vi "Set Topic Value.vi"(8 "error in (no error)":errorcluster, 9 "Value":variant, 10 "Topic":string, 11 "Communications in":refnum<class "Communications.lvclass">) -> (0 "error out":errorcluster, 2 "replaced":bool, 3 "Communications out":refnum<class "Communications.lvclass">)   [LabVIEW 2019, in "Communications.lvclass"]
uses:
  Communications.lvclass
  Communications.lvclass/Communications.ctl
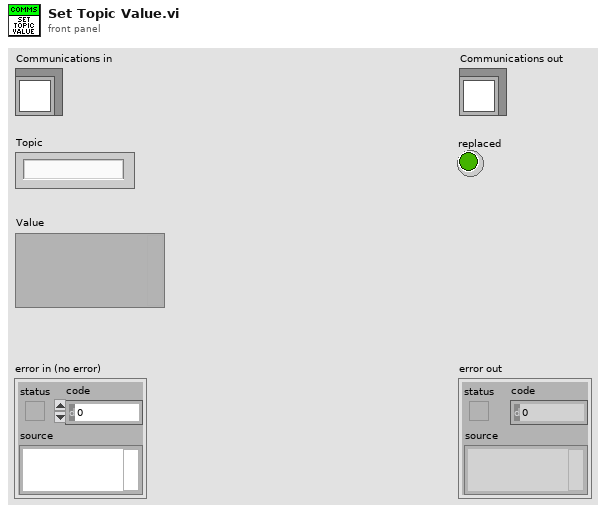
[diagram p1: front panel]
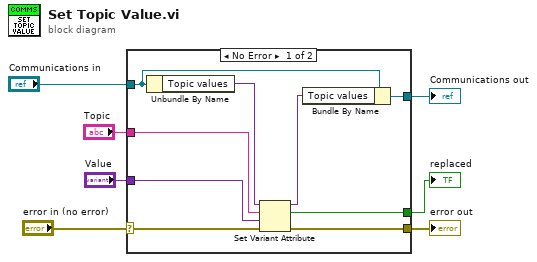
[diagram p0: block diagram]
diagram:
  n1 = case shown="No Error" "error in (no error)" {
    selector: "error in (no error)" -> [w14 w18]
    tunnel: [w11 w18] -> w6
    tunnel: [w10 w17] -> w4
    tunnel: "Communications in" -> [w16 w17]
    tunnel: "Value" -> [w13 _]
    tunnel: "Topic" -> [w12 _]
    tunnel: [w8 _] -> w1
    frame No Error {
      n2 = Unbundle By Name(w16) -> ("Topic values"=w15:variant)
      n3 = Set Variant Attribute(Variant=w15, name=w12, value=w13, error in=w14) -> (Variant out=w9:variant, replaced=w8:bool, error out=w11:errorcluster)
      n4 = Bundle By Name(cluster=w16, "Topic values"=w9) -> (w10:refnum<class "Communications.lvclass">)
    }
    frame Error {
    }
  }
  "error out" <- w6
  "Communications out" <- w4
  "replaced" <- w1
